vi "2086发送波浪仪.vi"(8 "columns":string[](array[string]), 9 "table":string, 10 "拆分数据":bool, 11 "data":string[][](array[string])) -> ()   [LabVIEW 2016, in "数据传输系统-03.lvlib"]
uses:
  <vilib>/Utility/config.llb/Write Key (String).vi
  <vilib>/Utility/config.llb/Read Key (String).vi
  <vilib>/Utility/config.llb/NI_LVConfig.lvlib
panel:
  out "数据拆分":bool
  out "数据发送起始时间":timestamp format="%<%.3X\n%Y/%m/%d>T"
  in  "设备类型":string(combo)="010200"
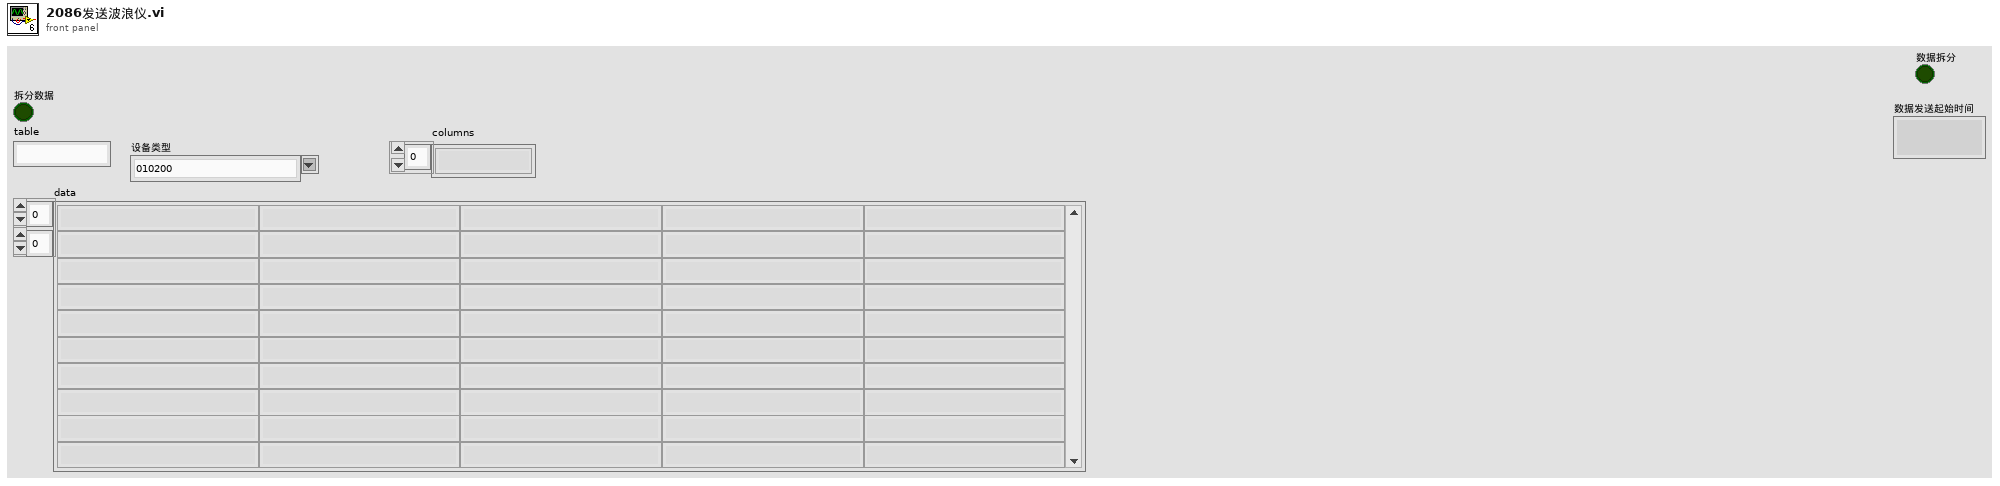
[diagram p1: front panel]
types:
  T1 = cluster{"QN":string, "ST":string, "CN":string, "PW":string, "MN":string, "FLAG":string, "PNUM":string, "PNO":string, "CP":string}
  T2 = typedef "LVComboBoxStrsAndValuesArrayTypeDef.ctl" = cluster{"String":string, "Value":string}[]
  T3 = typedef "数据传输系统-03.lvlib/应用环境.ctl" = enum16{"STD", "GB212", "婉仪平台"}
  T4 = cluster{"setini":string, "sysini":string, "hechaini":string, "actualwrite":string, "actualread":string, "datasent":string, "反控命令信息队列":string, "反控与仪器交互":string}
  T5 = typedef "NI_LVConfig.lvlib/Config Data RefNum.ctl" = refnum<k1>
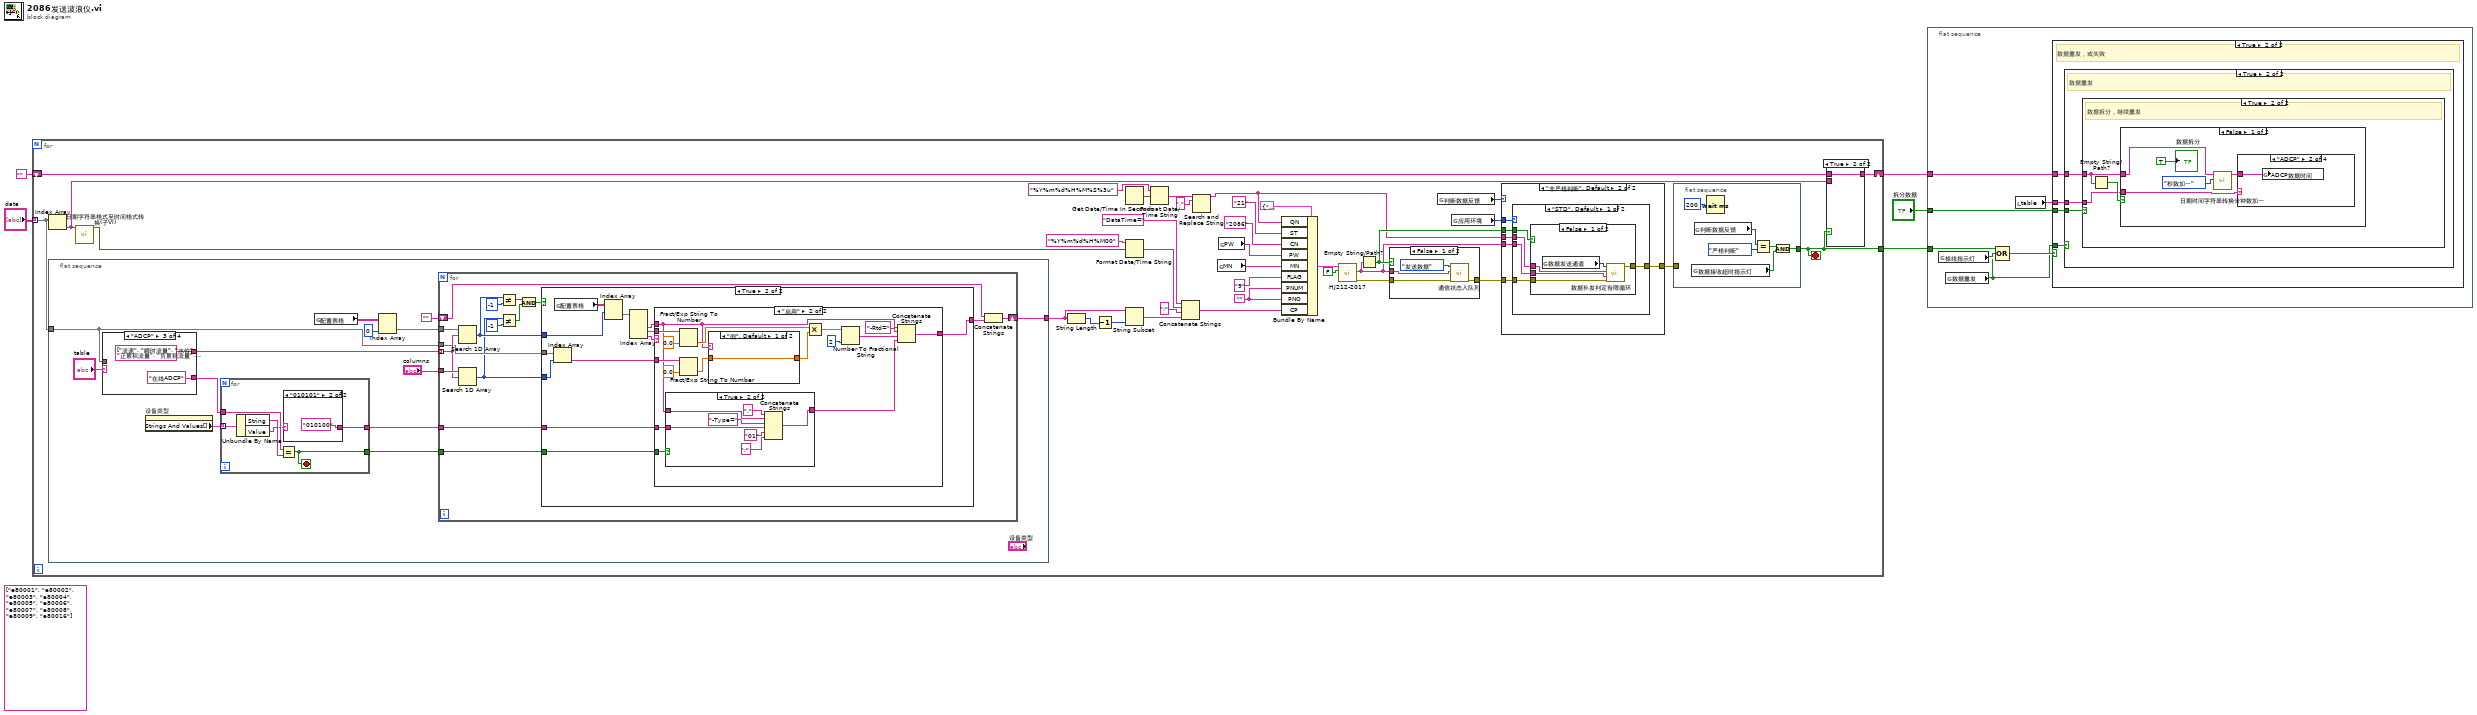
[diagram p0: block diagram]
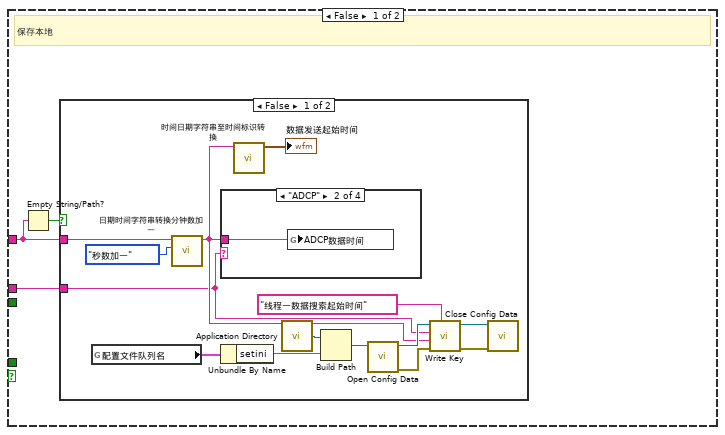
[diagram p2: hidden frame]
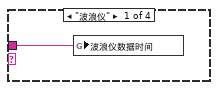
[diagram p3: hidden frame]
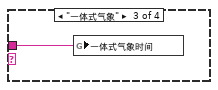
[diagram p4: hidden frame]
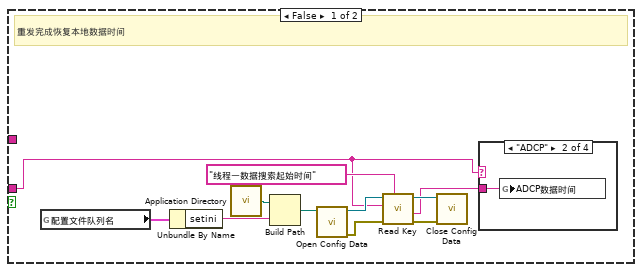
[diagram p8: hidden frame]
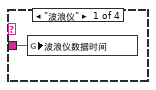
[diagram p9: hidden frame]
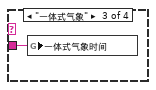
[diagram p10: hidden frame]
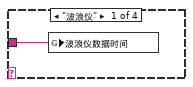
[diagram p12: hidden frame]
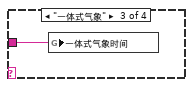
[diagram p13: hidden frame]
diagram:
  (unwired) string[] ["e80001", "e80002", "e80003", "e80004", "e80005", "e80006", "e80007", "e80008", "e80009", "e80016"] ("子数组")
  n1 = for {
    tunnel: "data" -> [w27] mode=indexing
    shift-right: [w14] -> w3
    shift-left: "" -> [w15]
    tunnel: [w13] -> w4
    stop <- w13 stop-if-true
    w31 = ""
    n2 = Index Array(array=w27) -> (element=w9:string)  [unwired: 1 in]
    n3 = flat-sequence {
      tunnel: w27 -> [w72]
      tunnel: [w75] -> w12
      frame #0 {
        n4 = case shown="\"ADCP\"" "table" {
          tunnel: [_ string[] ["空气温度", "相对湿度", "气压", "风速", "风向", "分钟雨量", "小时雨量", "日雨量", "累积雨量"] ("数组") string[] ["流速", "瞬时流量", "水位", "正累积流量", "负累积流量", "横摇", "纵摇", "电压"] ("数组") string[] ["最大波高", "最大波周期", "1/10波高", "1/10波周期", "有效波高", "有效波周期", "平均波高", "平均波周期", "波向", "波数"] ("数组")] -> w73
          tunnel: w72 -> [_ _ _ w89]
          tunnel: [_ "一体式气象仪" "在线ADCP" w88] -> w71
          frame "假", Default {
          }
          frame "一体式气象" {
          }
          frame "ADCP" {
          }
          frame "波浪仪" {
            n5 = Array Size(array=w89) -> (size(s)=w91:i32)
            n6 = Decrement(x=w91) -> (x-1=w90:i32)
            n7 = Index Array(array=w89, index=w90) -> (element=w88:string)
          }
        }
        n8 = property on="设备类型" class="CmbBox"() -> ("Strings And Values[]"=w83:T2)  [unwired: 2 in, 2 out]
        n9 = for {
          tunnel: w83 -> [w156] mode=indexing
          tunnel: w71 -> [w154]
          tunnel: [w151] -> w76
          tunnel: [w153] -> w77
          stop <- w153 stop-if-true
          n10 = Unbundle By Name(w156) -> ("String"=w155:string, "Value"=w152:string)
          n11 = Equal?(x=w154, y=w155) -> (x = y?=w153:bool)
          n12 = case shown="\"010101\"" w152 {
            selector: w152 -> [w157 _]
            tunnel: [w157 "010100" ("时间格式字符串(%c)")] -> w151
            frame "假", Default {
            }
            frame "010101" {
            }
          }
        }
        n13 = global read "断电保存全局.vi" "配置表格"() -> (w78:string[][])
        n14 = Index Array(array=w78, index (col)=0 ("禁用的索引 (列)")) -> (element=w80:string[])  [unwired: 1 in]
        n15 = for {
          tunnel: w80 -> [w108]
          tunnel: w73 -> [w102] mode=indexing
          tunnel: "columns" -> [w105]
          shift-right: [w98] -> w75
          shift-left: "" -> [w99]
          tunnel: w77 -> [w96]
          tunnel: w76 -> [w95]
          tunnel: w72 -> [w94]
          n16 = Search 1D Array(1D array=w108, element=w102) -> (index of element=w106:i32)  [unwired: 1 in]
          n17 = Search 1D Array(1D array=w105, element=w102) -> (index of element=w93:i32)  [unwired: 1 in]
          n18 = Not Equal?(x=w106, y=-1) -> (x != y?=w101:bool)
          n19 = Not Equal?(x=w93, y=-1) -> (x != y?=w103:bool)
          n20 = And(x=w101, y=w103) -> (x .and. y?=w100:bool)
          n21 = case shown="True" w100 {
            tunnel: w106 -> [_ w120]
            tunnel: ["" w115] -> w97
            tunnel: w96 -> [_ w114]
            tunnel: w95 -> [_ w113]
            tunnel: w94 -> [_ w112]
            tunnel: w93 -> [_ w111]
            frame False {
            }
            frame True {
              n22 = Index Array(array=w112, index=w111) -> (element=w110:string)
              n23 = global read "断电保存全局.vi" "配置表格"() -> (w121:string[][])
              n24 = Index Array(array=w121, index (row)=w120) -> (element=w119:string[])  [unwired: 1 in]
              n25 = Index Array(array=w119) -> (element #2=w117:string, element #3=w116:string, element #4=w118:string)  [unwired: 4 in, 1 out]
              n26 = case shown="\"启用\"" w118 {
                tunnel: w117 -> [_ w125]
                tunnel: w116 -> [_ w137]
                tunnel: ["" w134] -> w115
                tunnel: w114 -> [_ w133]
                tunnel: w113 -> [_ w132]
                tunnel: w110 -> [_ w130]
                frame "假", Default {
                }
                frame "启用" {
                  n27 = case shown="True" w133 {
                    tunnel: w125 -> [_ w150]
                    tunnel: w132 -> [_ w148]
                    tunnel: [";" ("字符串") w144] -> w135
                    frame False {
                    }
                    frame True {
                      n28 = Concatenate Strings("," ("字符串"), w150, "-Type=" ("格式字符串"), w148, "01" ("字符串"), ";" ("字符串")) -> (w144:string)
                    }
                  }
                  n29 = Fract/Exp String To Number(string=w137, default (0 dbl)=sgl 0.0 ("默认(0 DBL)")) -> (number=w129:sgl)  [unwired: 2 in, 1 out]
                  n30 = Fract/Exp String To Number(string=w130, default (0 dbl)=sgl 0.0 ("默认(0 DBL)")) -> (number=w124:sgl)  [unwired: 2 in, 1 out]
                  n31 = case shown="\"假\", Default" w125 {
                    tunnel: w124 -> [w139 w142]
                    tunnel: [w139 w140] -> w123
                    frame "假", Default {
                    }
                    frame "e01901" {
                      n32 = Divide(x=w142, y=sgl 1000.0) -> (x/y=w140:sgl)
                    }
                  }
                  n33 = Multiply(x=w129, y=w123) -> (x*y=w128:sgl)
                  n34 = Number To Fractional String(number=w128, precision (6)=i16 2 ("精度(6)")) -> (F-format string=w126:string)  [unwired: 2 in]
                  n35 = Concatenate Strings(w125, "-Rtd=" ("时间格式字符串(%c)"), w126, w135) -> (w134:string)
                }
              }
            }
          }
          n36 = Concatenate Strings(w99, w97) -> (w98:string)
        }
      }
    }
    n37 = call "日期字符串格式至时间格式转换(子VI).vi"("data[0]"=w9) -> ("time stamp"=w7:timestamp)  [unwired: 10 in]
    n38 = String Length(string=w12) -> (length=w26:i32)
    n39 = Decrement(x=w26) -> (x-1=w11:i32)
    n40 = Get Date/Time In Seconds() -> (seconds since 1Jan1904=w39:timestamp)
    n41 = Format Date/Time String(time format string (%c)="%Y%m%d%H%M00" ("时间格式字符串(%c)"), seconds (now)=w7) -> (date/time string=w6:string)  [unwired: 1 in]
    n42 = String Subset(string=w12, length (rest)=w11) -> (substring=w10:string)  [unwired: 1 in]
    n43 = Format Date/Time String(time format string (%c)="%Y%m%d%H%M%S%3u" ("时间格式字符串(%c)"), seconds (now)=w39) -> (date/time string=w38:string)  [unwired: 1 in]
    n44 = Concatenate Strings("DataTime=" ("时间格式字符串(%c)"), w6, ";" ("字符串"), w10) -> (w30:string)
    n45 = Search and Replace String(input string=w38, search string="." ("搜索字符串")) -> (result string=w17:string)  [unwired: 6 in, 3 out]
    n46 = global read "断电保存全局.vi" "MN"() -> (w36:string)
    n47 = global read "断电保存全局.vi" "PW"() -> (w35:string)
    n48 = Bundle By Name(cluster=T1 {"QN"="", "ST"="", "CN"="", "PW"="", "MN"="", "FLAG"="", "PNUM"="", "PNO"="", "CP"=""} ("数据块"), "QN"=w17, "ST"="21", "CN"="2086", "PW"=w35, "MN"=w36, "FLAG"="9", "PNUM"=w31, "PNO"=w31, "CP"=w30) -> (w18:T1)
    n49 = call "HJ212-2017.vi"("PWD？"=FALSE, "数据段"=w18) -> ("error out"=w19:errorcluster, "通讯包字符串"=w20:string)  [unwired: 7 in, 1 out]
    n50 = Empty String/Path?(string/path=w20) -> (empty?=w24:bool)
    n51 = case shown="False" w24 {
      tunnel: [w53 w54] -> w22
      tunnel: w19 -> [w52 w54]
      tunnel: w20 -> [w50 _]
      frame False {
        n52 = call "通信状态入队列.vi"("错误输入（无错误）"=w52, "发送报文"=w50, "枚举"=enum16{"打开连接", "发送数据", "读取数据", "数据处理", "关闭连接"}."发送数据") -> ("错误输出"=w53:errorcluster)  [unwired: 8 in]
      }
      frame True {
      }
    }
    n53 = global read "断电保存全局.vi" "判断数据反馈"() -> (w21:enum16{"非严格判断", "严格判断", "不判断"})
    n54 = global read "断电保存全局.vi" "应用环境"() -> (w23:T3)
    n55 = case shown="\"非严格判断\", Default" w21 {
      tunnel: w20 -> [_ w60]
      tunnel: w22 -> [_ w59]
      tunnel: w17 -> [_ w58]
      tunnel: w23 -> [_ w57]
      tunnel: w24 -> [_ w56]
      tunnel: [_ w55] -> w16
      frame "不判断" {
      }
      frame "非严格判断", Default {
        n56 = case shown="\"STD\", Default" w57 {
          tunnel: w60 -> [w63 _]
          tunnel: w59 -> [w65 _]
          tunnel: w58 -> [w64 _]
          tunnel: w56 -> [w62 _]
          tunnel: [w61 _] -> w55
          frame "STD", Default {
            n57 = case shown="False" w62 {
              tunnel: w65 -> [w70 _]
              tunnel: w64 -> [w68 _]
              tunnel: w63 -> [w67 _]
              tunnel: [w66 _] -> w61
              frame False {
                n58 = global read "断电保存全局.vi" "数据发送通道"() -> (w69:enum16{"TCP", "VISA"})
                n59 = call "数据补发判定有限循环.vi"("错误输入（无错误）"=w70, "数据输入"=w67, "QN"=w68, "数据发送通道"=w69) -> ("error out"=w66:errorcluster)  [unwired: 7 in]
              }
              frame True {
              }
            }
          }
          frame "GB212" {
          }
        }
      }
    }
    n60 = flat-sequence {
      tunnel: [w46] -> w13
      tunnel: w16 -> [_]
      frame #0 {
        n61 = global read "全局 数据发送重叠.vi" "数据接收超时指示灯"() -> (w49:bool)
        n62 = global read "断电保存全局.vi" "判断数据反馈"() -> (w47:enum16{"非严格判断", "严格判断", "不判断"})
        n63 = Wait (ms)(milliseconds to wait=u32 200 ("等待时间（毫秒）")) -> ()  [unwired: 1 out]
        n64 = Equal?(x=w47, y=enum16{"非严格判断", "严格判断", "不判断"}."严格判断") -> (x = y?=w44:bool)
        n65 = And(x=w44, y=w49) -> (x .and. y?=w46:bool)
      }
    }
    n66 = case shown="True" w13 {
      tunnel: w15 -> [_ w43]
      tunnel: [w42 w43] -> w14
      tunnel: w9 -> [w42 _]
      frame False {
      }
      frame True {
      }
    }
  }
  n67 = flat-sequence {
    tunnel: w4 -> [w162]
    tunnel: w3 -> [w161]
    tunnel: "拆分数据" -> [w160]
    frame #0 {
      n68 = global read "全局 数据发送重叠.vi" "掉线指示灯"() -> (w165:bool)
      n69 = global read "断电保存全局.vi" "数据重发"() -> (w163:bool)
      n70 = Compound Arithmetic op=OR ("复合运算")(w162, w165, w163) -> (w164:bool)
      n71 = local read "table"() -> (w159:string)
      n72 = case shown="True" w164 {
        tunnel: w161 -> [w166 w186]
        tunnel: w159 -> [w168 w189]
        tunnel: w163 -> [_ w188]
        tunnel: w160 -> [_ w187]
        frame False {
          # "保存本地"
          n73 = Empty String/Path?(string/path=w166) -> (empty?=w167:bool)
          n74 = case shown="False" w167 {
            tunnel: w168 -> [w169 _]
            tunnel: w166 -> [w171 _]
            frame False {
              n75 = global read "全局1.vi" "配置文件队列名"() -> (w172:T4)
              n76 = call "日期时间字符串转换分钟数加一.vi"("枚举"=enum16{"分钟数加一", "秒数加一", "小时数加一"}."秒数加一", "data[0]"=w171) -> ("日期/时间字符串"=w170:string)  [unwired: 9 in]
              n77 = case shown="\"ADCP\"" w169 {
                tunnel: w170 -> [w183 w184 w185 _]
                frame "波浪仪" {
                  n78 = global write "全局 水样时间.vi" "波浪仪数据时间"(w183) -> ()
                }
                frame "ADCP" {
                  n79 = global write "全局 水样时间.vi" "ADCP数据时间"(w184) -> ()
                }
                frame "一体式气象" {
                  n80 = global write "全局 水样时间.vi" "一体式气象时间"(w185) -> ()
                }
                frame "假", Default {
                }
              }
              n81 = Unbundle By Name(w172) -> ("setini"=w173:string)
              n82 = call "时间日期字符串至时间标识转换.vi"("时间日期字符串"=w170) -> ("时间标识"=→"数据发送起始时间":timestamp)  [unwired: 10 in]
              n83 = call <vilib>:"Application Directory.vi"() -> ("Application Directory"=w176:path)
              n84 = Build Path(base path=w176, name or relative path=w173) -> (appended path=w177:path)
              n85 = call <vilib>:"Open Config Data.vi"("configuration file path"=w177) -> ("error out"=w179:errorcluster, "refnum"=w178:T5)  [unwired: 8 in, 1 out]
              n86 = call-poly <vilib>:"Write Key.vi"("section"="线程一数据搜索起始时间", "error in (no error)"=w179, "value"=w170, "key"=w169, "refnum"=w178) -> ("error out"=w181:errorcluster, "refnum out"=w180:T5)  [unwired: 4 in, 1 out]
              n87 = call <vilib>:"Close Config Data.vi"("error in (no error)"=w181, "refnum"=w180) -> ()  [unwired: 8 in, 2 out]
            }
            frame True {
            }
          }
        }
        frame True {
          # "数据重发，或失败"
          n88 = case shown="True" w188 {
            tunnel: w189 -> [_ w192]
            tunnel: w187 -> [_ w191]
            tunnel: w186 -> [_ w190]
            frame False {
              # "数据发送失败"
            }
            frame True {
              # "数据重发"
              n89 = case shown="True" w191 {
                tunnel: w192 -> [w194 w207]
                tunnel: w190 -> [_ w208]
                frame False {
                  # "重发完成恢复本地数据时间"
                  n90 = global read "全局1.vi" "配置文件队列名"() -> (w195:T4)
                  n91 = Unbundle By Name(w195) -> ("setini"=w202:string)
                  n92 = call <vilib>:"Application Directory.vi"() -> ("Application Directory"=w196:path)
                  n93 = Build Path(base path=w196, name or relative path=w202) -> (appended path=w197:path)
                  n94 = call <vilib>:"Open Config Data.vi"("configuration file path"=w197) -> ("error out"=w203:errorcluster, "refnum"=w198:T5)  [unwired: 8 in, 1 out]
                  n95 = call-poly <vilib>:"Read Key.vi"("section"="线程一数据搜索起始时间", "error in (no error)"=w203, "key"=w194, "refnum"=w198) -> ("error out"=w201:errorcluster, "value"=w193:string, "refnum out"=w200:T5)  [unwired: 4 in, 1 out]
                  n96 = call <vilib>:"Close Config Data.vi"("error in (no error)"=w201, "refnum"=w200) -> ()  [unwired: 8 in, 2 out]
                  n97 = case shown="\"ADCP\"" w194 {
                    tunnel: w193 -> [w204 w205 w206 _]
                    frame "波浪仪" {
                      n98 = global write "全局 水样时间.vi" "波浪仪数据时间"(w204) -> ()
                    }
                    frame "ADCP" {
                      n99 = global write "全局 水样时间.vi" "ADCP数据时间"(w205) -> ()
                    }
                    frame "一体式气象" {
                      n100 = global write "全局 水样时间.vi" "一体式气象时间"(w206) -> ()
                    }
                    frame "假", Default {
                    }
                  }
                }
                frame True {
                  # "数据拆分，继续重发"
                  n101 = Empty String/Path?(string/path=w208) -> (empty?=w209:bool)
                  n102 = case shown="False" w209 {
                    tunnel: w208 -> [w212 _]
                    tunnel: w207 -> [w210 _]
                    frame False {
                      n103 = call "日期时间字符串转换分钟数加一.vi"("枚举"=enum16{"分钟数加一", "秒数加一", "小时数加一"}."秒数加一", "data[0]"=w212) -> ("日期/时间字符串"=w211:string)  [unwired: 9 in]
                      n104 = case shown="\"ADCP\"" w210 {
                        tunnel: w211 -> [w215 w216 w217 _]
                        frame "波浪仪" {
                          n105 = global write "全局 水样时间.vi" "波浪仪数据时间"(w215) -> ()
                        }
                        frame "ADCP" {
                          n106 = global write "全局 水样时间.vi" "ADCP数据时间"(w216) -> ()
                        }
                        frame "一体式气象" {
                          n107 = global write "全局 水样时间.vi" "一体式气象时间"(w217) -> ()
                        }
                        frame "假", Default {
                        }
                      }
                      "数据拆分" <- TRUE
                    }
                    frame True {
                    }
                  }
                }
              }
            }
          }
        }
      }
    }
  }
